vi "Calculate Center.vi"(10 "Relative Coordinates":dbl[][](array[numeric]), 11 "Fiducial Measurements":dbl[][](array[numeric])) -> (3 "XYZTheta Centers":dbl[][](array[numeric]))   [LabVIEW 2019, in "Pick Up Tool Fixture.lvclass"]
uses:
  Pick Up Tool Fixture.lvclass
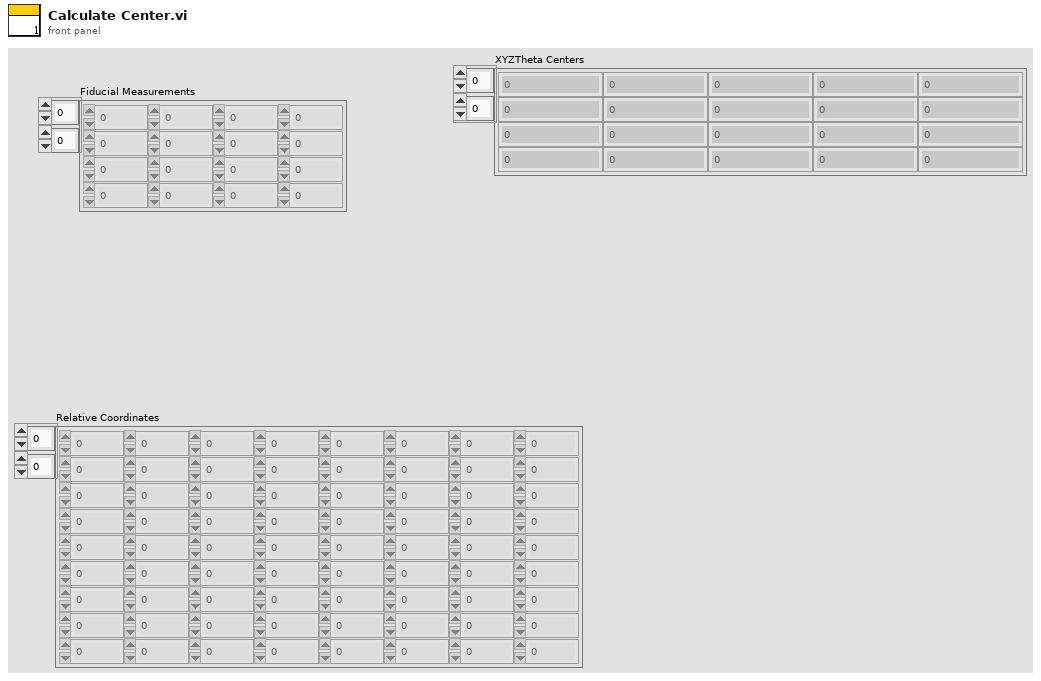
[diagram p1: front panel]
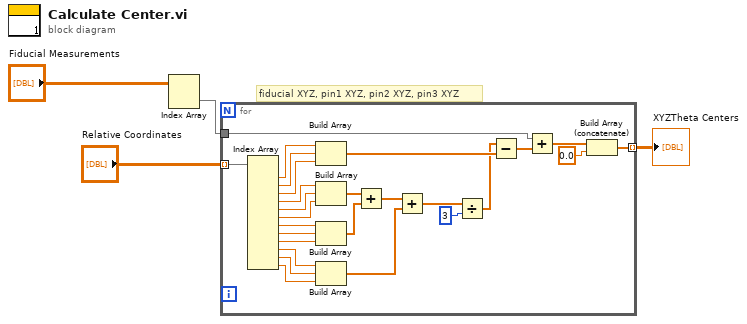
[diagram p0: block diagram]
diagram:
  # "fiducial XYZ, pin1 XYZ, pin2 XYZ, pin3 XYZ"
  n1 = Index Array(array="Fiducial Measurements") -> (element=w2:dbl[])  [unwired: 2 in]
  n2 = for {
    tunnel: "Relative Coordinates" -> [w28] mode=indexing
    tunnel: w2 -> [w8]
    tunnel: [w5] -> w1 mode=indexing
    n3 = Index Array(array=w28) -> (element #1=w30:dbl, element #2=w29:dbl, element #3=w12:dbl, element #4=w27:dbl, element #5=w26:dbl, element #6=w25:dbl, element #7=w24:dbl, element #8=w23:dbl, element #9=w22:dbl, element #10=w21:dbl, element #11=w20:dbl, element #12=w19:dbl)  [unwired: 12 in]
    n4 = Build Array(w30, w29, w12) -> (w11:dbl[])
    n5 = Build Array(w27, w26, w25) -> (w18:dbl[])
    n6 = Build Array(w24, w23, w22) -> (w17:dbl[])
    n7 = Build Array(w21, w20, w19) -> (w15:dbl[])
    n8 = Add(x=w18, y=w17) -> (x+y=w16:dbl[])
    n9 = Add(x=w16, y=w15) -> (x+y=w14:dbl[])
    n10 = Divide(x=w14, y=3) -> (x/y=w10:dbl[])
    n11 = Subtract(x=w10, y=w11) -> (x-y=w9:dbl[])
    n12 = Add(x=w8, y=w9) -> (x+y=w7:dbl[])
    n13 = Build Array (concatenate)(w7, 0.0) -> (w5:dbl[])
  }
  "XYZTheta Centers" <- w1
